vi "Data Logger Global Variable.vi"() -> ()   [LabVIEW 2014]
uses:
  <vilib>/Utility/miscctls.llb/LVPointTypeDef.ctl
  <vilib>/Utility/miscctls.llb/LVRectTypeDef.ctl
panel:
  in  "FP Bounds":T1={"Left"=105, "Top"=-7, "Right"=1816, "Bottom"=994}
  in  "Active Display":u16
  in  "Pane Origin":T2[](array[typedef])
  in  "System Tray":enum16{"Enabled", "Disabled"}(ring)
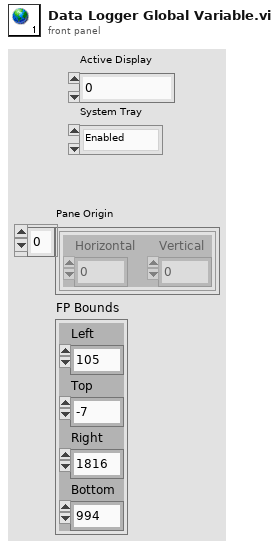
[diagram p1: front panel]
types:
  T1 = typedef "LVRectTypeDef.ctl" = cluster{"Left":i16, "Top":i16, "Right":i16, "Bottom":i16}
  T2 = typedef "LVPointTypeDef.ctl" = cluster{"Horizontal":i16, "Vertical":i16}
diagram:
